vi "measurement sweep.vi"(6 "Delta H (mT)":dbl=0.5, 7 "const phi?":bool=TRUE, 8 "error in (no error)":errorcluster, 9 "delta phi (deg)":dbl=0.5, 10 "sweep parameter":T1=enum."magnetic field", 11 "magnet initial":T3) -> (0 "error out":errorcluster, 3 "measdata definition":T2 {"Current Magnetic\nField\n(430 TCP reading)"."phi (deg)" format="%#_3g"})   [LabVIEW 2013]
uses:
  devices/magnet/magnet polar field.ctl
  measdata cluster.ctl
  measurement sweep parameter.ctl
  devices/magnet/AMI reading polar field.ctl
  config.vi
panel:
  # "List of measurement data for the S-parameters."
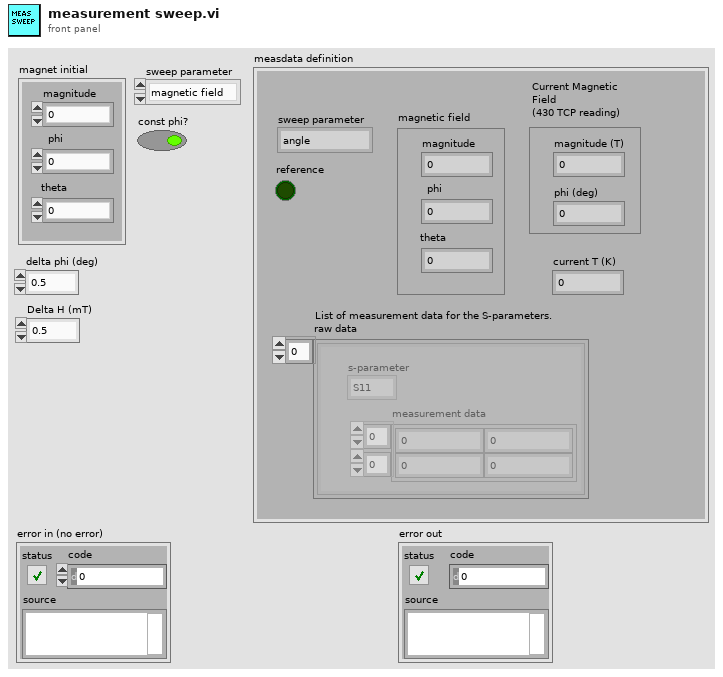
[diagram p1: front panel]
types:
  T1 = typedef "measurement sweep parameter.ctl" = enum16{"angle", "magnetic field"}
  T2 = typedef "measdata cluster.ctl" = cluster{"raw data":cluster{"measurement data":dbl[][], "s-parameter":enum16{"S11", "S12", "S21", "S22"}}[], "magnetic field":T3, "reference":bool, "sweep parameter":T1, "Current Magnetic\nField\n(430 TCP reading)":T4, "current T (K)":dbl}
  T3 = typedef "magnet polar field.ctl" = cluster{"magnitude":dbl, "phi":dbl, "theta":dbl}
  T4 = typedef "AMI reading polar field.ctl" = cluster{"magnitude (T)":dbl, "phi (deg)":dbl}
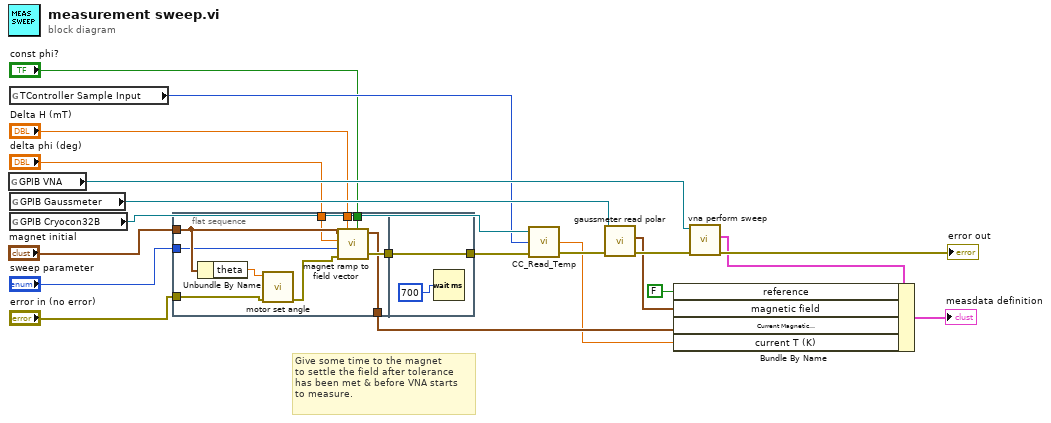
[diagram p0: block diagram]
diagram:
  # "Give some time to the magnet \nto settle the field after tolerance\nhas been met & before VNA starts\nto measure."
  n1 = global read "config.vi" "GPIB VNA"() -> (w15:refnum<visa-resource-name>)
  n2 = global read "config.vi" "TController Sample Input"() -> (w8:u8)
  n3 = global read "config.vi" "GPIB Gaussmeter"() -> (w16:refnum<visa-resource-name>)
  n4 = global read "config.vi" "GPIB Cryocon32B"() -> (w11:refnum<visa-resource-name>)
  n5 = flat-sequence {
    tunnel: [w26] -> w13
    tunnel: "magnet initial" -> [w29]
    tunnel: "error in (no error)" -> [w31]
    tunnel: [w27] -> w6
    tunnel: "sweep parameter" -> [w25]
    tunnel: "const phi?" -> [w24]
    tunnel: "Delta H (mT)" -> [w23]
    tunnel: "delta phi (deg)" -> [w22]
    tunnel: [w33] -> w10
    tunnel: w6 -> [w33]
    frame #0 {
      n6 = Unbundle By Name(w29) -> ("theta"=w30:dbl)
      n7 = call "motor set angle.vi"("error in (no error)"=w31, "angle"=w30) -> ("error out"=w28:errorcluster)  [unwired: 9 in]
      n8 = call "magnet ramp to field vector.vi"("const phi?"=w24, "Delta H (mT)"=w23, "error in (no error)"=w28, "sweep parameter"=w25, "delta phi (deg)"=w22, "magnet polar"=w29) -> ("error out"=w27:errorcluster, "Current Magnetic\nField\n(430 TCP reading)"=w26:T4)  [unwired: 3 in]
    }
    frame #1 {
      n9 = Wait (ms)(milliseconds to wait=u32 700) -> ()  [unwired: 1 out]
    }
  }
  n10 = call <userlib>:"CC_Read_Temp.vi"("error in (no error)"=w10, "Input"=w8, "VISA In"=w11) -> ("error out"=w9:errorcluster, "Temperature"=w7:dbl)  [unwired: 1 out]
  n11 = call "gaussmeter read polar.vi"("error in (no error)"=w9, "VISA resource name"=w16) -> ("error out"=w20:errorcluster, "magnet polar"=w14:T3)  [unwired: 7 in, 1 out]
  n12 = call "vna perform sweep.vi"("error in (no error)"=w20, "VISA resource name"=w15) -> ("error out"=→"error out":errorcluster, "measdata definition"=w17:T2)  [unwired: 7 in, 1 out]
  n13 = Bundle By Name(cluster=w17, "reference"=FALSE, "magnetic field"=w14, "Current Magnetic\nField\n(430 TCP reading)"=w13, "current T (K)"=w7) -> (→"measdata definition":T2)
